vi "listTestMethods.vi"(10 "Methods":path[](array[path])) -> (1 "Test Method Names":string[](array[string]), 2 "Test Method Paths":path[](array[path]))   [LabVIEW 2013, in "TestLoader.lvclass"]
uses:
  TestLoader.lvclass
  <userlib>/_OpenG.lib/array/array.llb/Conditional Auto-Indexing Tunnel (Path)__ogtk.vi
  <userlib>/_OpenG.lib/array/array.llb/Conditional Auto-Indexing Tunnel (String)__ogtk.vi
  <userlib>/_OpenG.lib/file/file.llb/Strip Path Extension - String__ogtk.vi
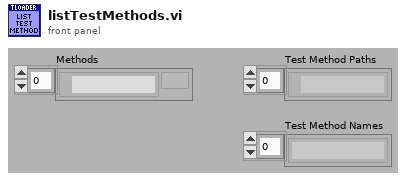
[diagram p1: front panel]
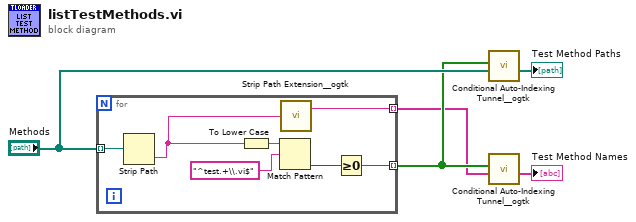
[diagram p0: block diagram]
diagram:
  n1 = for {
    tunnel: [w9] -> w3 mode=indexing
    tunnel: "Methods" -> [w8] mode=indexing
    tunnel: [w6] -> w1 mode=indexing
    n2 = Strip Path(path=w8) -> (name=w7:string)  [unwired: 1 out]
    n3 = To Lower Case(string=w7) -> (all lower case string=w12:string)
    n4 = Match Pattern(string=w12, regular expression="^test.+\\.vi$") -> (offset past match=w10:i32)  [unwired: 1 in, 3 out]
    n5 = call-poly <userlib>:"Strip Path Extension__ogtk.vi"("path"=w7) -> ("root"=w6:string)  [unwired: 1 out]
    n6 = Greater Or Equal To 0?(x=w10) -> (x >= 0?=w9:bool)
  }
  n7 = call-poly <userlib>:"Conditional Auto-Indexing Tunnel__ogtk.vi"("Array in"="Methods", "Elements to keep"=w3) -> ("Filtered Array out"=→"Test Method Paths":path[])  [unwired: 5 in]
  n8 = call-poly <userlib>:"Conditional Auto-Indexing Tunnel__ogtk.vi"("Array in"=w1, "Elements to keep"=w3) -> ("Filtered Array out"=→"Test Method Names":string[])  [unwired: 5 in]
